vi "VI Tree.vi"   [LabVIEW 2018, in "Agilent PSG MXG Series.lvlib"]
doc: "This is the instrument driver for the Agilent PSG MXG Series. The VI Tree displays all the user-callable VIs of the instrument driver in an organized table."
uses:
  Agilent PSG MXG Series.lvlib
  Configure/Modulation/Configure Modulation (Amplitude).vi
  Configure/Modulation/Configure Modulation Waveform (Noise).vi
  Configure/Configure Sweep (List).vi
  Configure/Modulation/Configure Modulation Waveform Advanced (Swept-Sine).vi
  Action-Status/Load and Save Data (Generic Data).vi
  Action-Status/Query Waveform Completed (Dual ARB).vi
panel:
  # "(c) 2007-2016 National Instruments.  ALL RIGHTS RESERVED."
  # "SEE DIAGRAM\nFOR VI TREE."
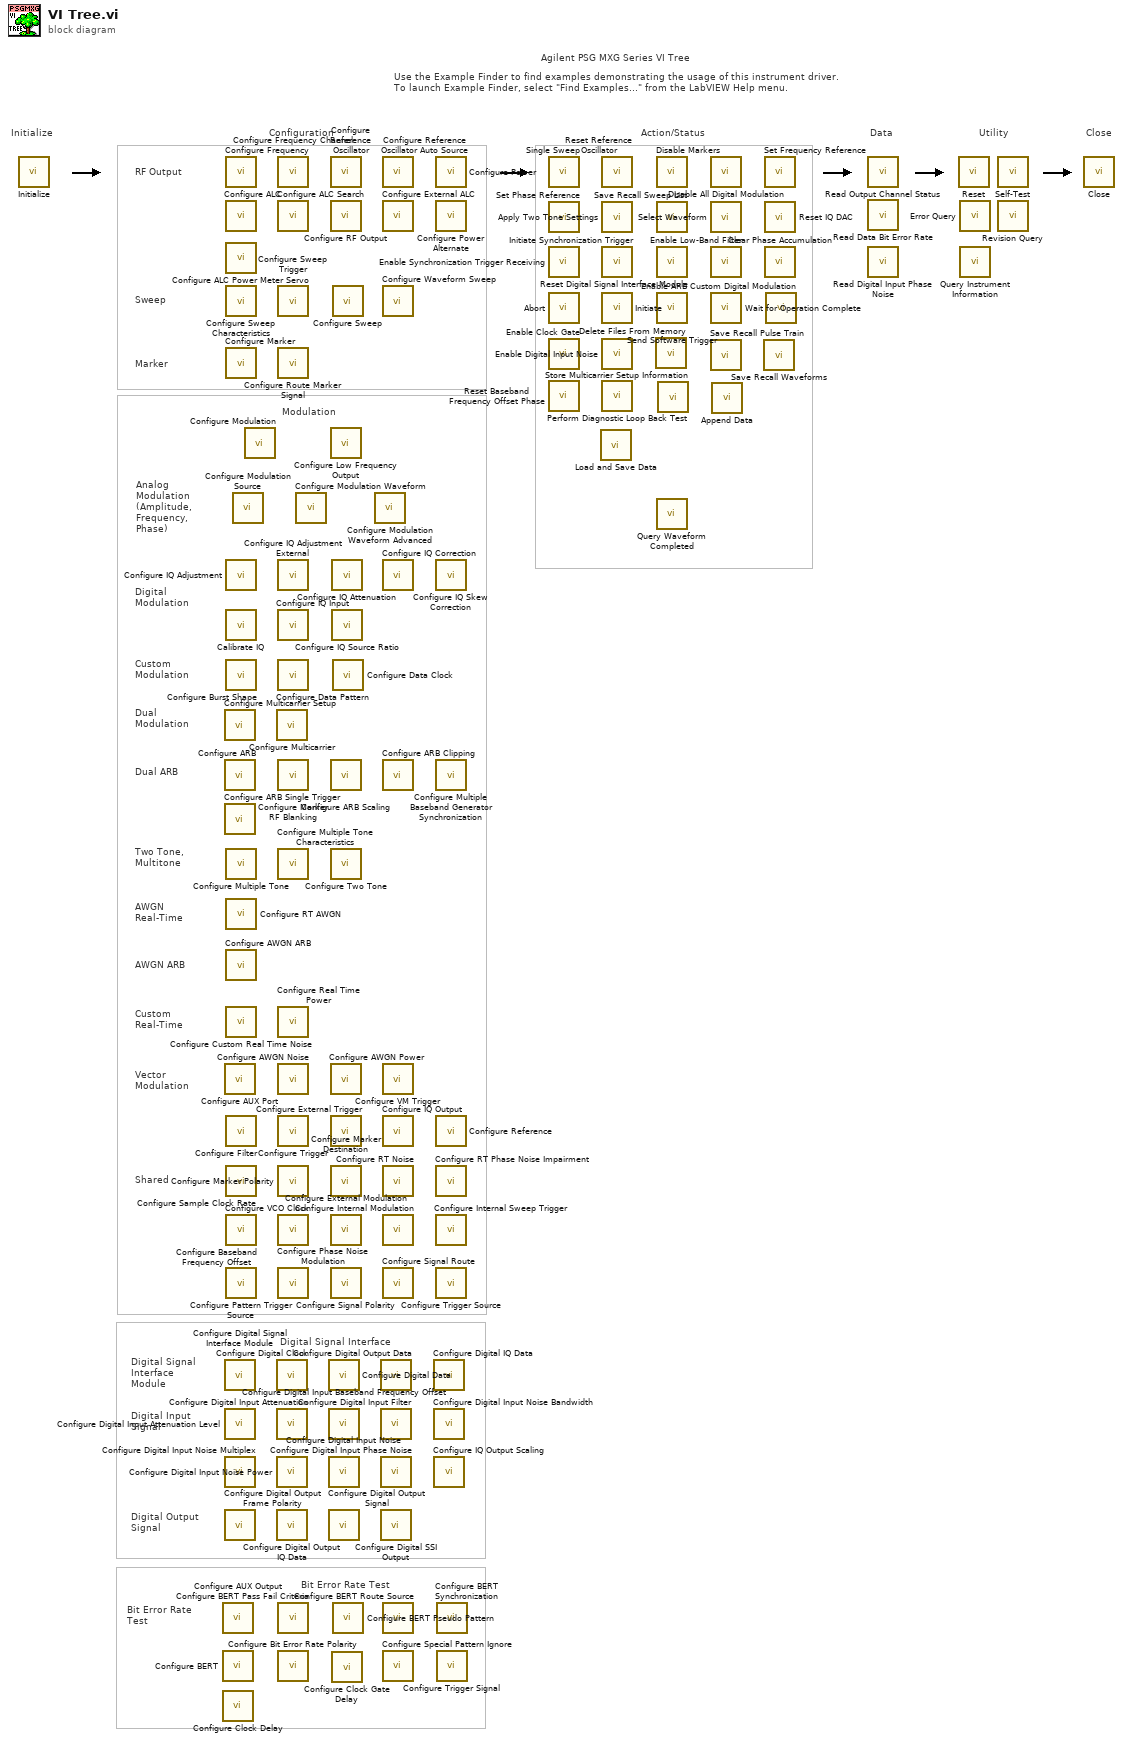
[diagram p0: block diagram]
diagram:
  # "Bit Error Rate Test"
  # "Bit Error Rate \nTest"
  # "Digital Output \nSignal"
  # "Digital Input \nSignal"
  # "Data"
  # "Vector\nModulation"
  # "Custom\nReal-Time"
  # "AWGN ARB"
  # "Digital Signal Interface"
  # "Marker"
  # "Digital Signal\nInterface\nModule"
  # "AWGN\nReal-Time"
  # "Shared"
  # "Two Tone,\nMultitone"
  # "Dual ARB"
  # "Dual\nModulation"
  # "Custom\nModulation"
  # "Digital\nModulation"
  # "Analog\nModulation\n(Amplitude,\nFrequency,\nPhase)"
  # "Sweep"
  # "RF Output"
  # "Modulation"
  # "Agilent PSG MXG Series VI Tree"
  # "Use the Example Finder to find examples demonstrating the usage of this instrument driver.\nTo launch Example Finder, select \"Find Examples...\" from the LabVIEW Help menu."
  # "Configuration"
  # "Utility"
  # "Action/Status"
  # "Close"
  # "Initialize"
  n1 = call "Initialize.vi"() -> ()  [unwired: 10 in, 2 out]
  n2 = call "Configure AUX Output.vi"() -> ()  [unwired: 10 in, 2 out]
  n3 = call "Configure BERT.vi"() -> ()  [unwired: 10 in, 2 out]
  n4 = call "Configure Clock Delay.vi"() -> ()  [unwired: 10 in, 2 out]
  n5 = call "Configure Multicarrier Setup.vi"() -> ()  [unwired: 14 in, 2 out]
  n6 = call "Configure ARB.vi"() -> ()  [unwired: 10 in, 2 out]
  n7 = call "Configure ARB Single Trigger.vi"() -> ()  [unwired: 10 in, 2 out]
  n8 = call "Configure AUX Port.vi"() -> ()  [unwired: 10 in, 2 out]
  n9 = call "Configure Digital Signal Interface Module.vi"() -> ()  [unwired: 10 in, 2 out]
  n10 = call "Configure Digital Input Attenuation Level.vi"() -> ()  [unwired: 10 in, 2 out]
  n11 = call "Configure Digital Input Noise Multiplex.vi"() -> ()  [unwired: 10 in, 2 out]
  n12 = call "Configure Digital Output Frame Polarity.vi"() -> ()  [unwired: 10 in, 2 out]
  n13 = call "Configure Frequency.vi"() -> ()  [unwired: 14 in, 2 out]
  n14 = call "Configure ALC.vi"() -> ()  [unwired: 14 in, 2 out]
  n15 = call "Configure ALC Power Meter Servo.vi"() -> ()  [unwired: 14 in, 2 out]
  n16 = call "Configure Sweep Characteristics.vi"() -> ()  [unwired: 14 in, 2 out]
  n17 = call "Configure Marker.vi"() -> ()  [unwired: 14 in, 2 out]
  n18 = call "Configure IQ Adjustment.vi"() -> ()  [unwired: 14 in, 2 out]
  n19 = call "Calibrate IQ.vi"() -> ()  [unwired: 10 in, 2 out]
  n20 = call "Configure Burst Shape.vi"() -> ()  [unwired: 14 in, 2 out]
  n21 = call "Configure Multiple Tone.vi"() -> ()  [unwired: 14 in, 2 out]
  n22 = call "Configure RT AWGN.vi"() -> ()  [unwired: 10 in, 2 out]
  n23 = call "Configure AWGN ARB.vi"() -> ()  [unwired: 10 in, 2 out]
  n24 = call "Configure Custom Real Time Noise.vi"() -> ()  [unwired: 10 in, 2 out]
  n25 = call "Configure Filter.vi"() -> ()  [unwired: 14 in, 2 out]
  n26 = call "Configure Sample Clock Rate.vi"() -> ()  [unwired: 10 in, 2 out]
  n27 = call "Configure Baseband Frequency Offset.vi"() -> ()  [unwired: 10 in, 2 out]
  n28 = call "Configure Pattern Trigger Source.vi"() -> ()  [unwired: 10 in, 2 out]
  n29 = call "Configure Modulation Source.vi"() -> ()  [unwired: 14 in, 2 out]
  n30 = call-poly "Configure Modulation.vi"() -> ()  [unwired: 14 in, 2 out]
  n31 = call "Configure Multicarrier.vi"() -> ()  [unwired: 10 in, 2 out]
  n32 = call "Configure Digital Clock.vi"() -> ()  [unwired: 14 in, 2 out]
  n33 = call "Configure Digital Input Attenuation.vi"() -> ()  [unwired: 10 in, 2 out]
  n34 = call "Configure Digital Input Noise Power.vi"() -> ()  [unwired: 10 in, 2 out]
  n35 = call "Configure Digital Output IQ Data.vi"() -> ()  [unwired: 10 in, 2 out]
  n36 = call "Configure Frequency Channel.vi"() -> ()  [unwired: 10 in, 2 out]
  n37 = call "Configure ALC Search.vi"() -> ()  [unwired: 14 in, 2 out]
  n38 = call "Configure Sweep Trigger.vi"() -> ()  [unwired: 14 in, 2 out]
  n39 = call "Configure Route Marker Signal.vi"() -> ()  [unwired: 10 in, 2 out]
  n40 = call "Configure IQ Adjustment External.vi"() -> ()  [unwired: 14 in, 2 out]
  n41 = call "Configure IQ Input.vi"() -> ()  [unwired: 10 in, 2 out]
  n42 = call "Configure Data Pattern.vi"() -> ()  [unwired: 10 in, 2 out]
  n43 = call "Configure Marker RF Blanking.vi"() -> ()  [unwired: 10 in, 2 out]
  n44 = call "Configure Multiple Tone Characteristics.vi"() -> ()  [unwired: 10 in, 2 out]
  n45 = call "Configure Real Time Power.vi"() -> ()  [unwired: 10 in, 2 out]
  n46 = call "Configure AWGN Noise.vi"() -> ()  [unwired: 14 in, 2 out]
  n47 = call "Configure Trigger.vi"() -> ()  [unwired: 14 in, 2 out]
  n48 = call "Configure Marker Polarity.vi"() -> ()  [unwired: 10 in, 2 out]
  n49 = call "Configure VCO Clock.vi"() -> ()  [unwired: 10 in, 2 out]
  n50 = call "Configure Phase Noise Modulation.vi"() -> ()  [unwired: 10 in, 2 out]
  n51 = call "Configure BERT Pass Fail Criteria.vi"() -> ()  [unwired: 10 in, 2 out]
  n52 = call "Configure Bit Error Rate Polarity.vi"() -> ()  [unwired: 10 in, 2 out]
  n53 = call-poly "Configure Modulation Waveform.vi"() -> ()  [unwired: 10 in, 2 out]
  n54 = call "Configure Digital Data.vi"() -> ()  [unwired: 14 in, 2 out]
  n55 = call "Configure Digital Input Baseband Frequency Offset.vi"() -> ()  [unwired: 10 in, 2 out]
  n56 = call "Configure Digital Input Noise.vi"() -> ()  [unwired: 10 in, 2 out]
  n57 = call "Configure Digital Output Signal.vi"() -> ()  [unwired: 10 in, 2 out]
  n58 = call "Configure Reference Oscillator.vi"() -> ()  [unwired: 10 in, 2 out]
  n59 = call "Configure RF Output.vi"() -> ()  [unwired: 10 in, 2 out]
  n60 = call "Configure Low Frequency Output.vi"() -> ()  [unwired: 14 in, 2 out]
  n61 = call "Configure ARB Scaling.vi"() -> ()  [unwired: 10 in, 2 out]
  n62 = call "Configure Two Tone.vi"() -> ()  [unwired: 10 in, 2 out]
  n63 = call "Configure AWGN Power.vi"() -> ()  [unwired: 10 in, 2 out]
  n64 = call "Configure External Trigger.vi"() -> ()  [unwired: 10 in, 2 out]
  n65 = call "Configure Marker Destination.vi"() -> ()  [unwired: 10 in, 2 out]
  n66 = call "Configure External Modulation.vi"() -> ()  [unwired: 10 in, 2 out]
  n67 = call "Configure Signal Polarity.vi"() -> ()  [unwired: 10 in, 2 out]
  n68 = call "Configure IQ Attenuation.vi"() -> ()  [unwired: 10 in, 2 out]
  n69 = call "Configure IQ Source Ratio.vi"() -> ()  [unwired: 10 in, 2 out]
  n70 = call "Configure Clock Gate Delay.vi"() -> ()  [unwired: 10 in, 2 out]
  n71 = call-poly "Configure Sweep.vi"() -> ()  [unwired: 14 in, 2 out]
  n72 = call "Configure Data Clock.vi"() -> ()  [unwired: 10 in, 2 out]
  n73 = call "Configure BERT Pseudo Pattern.vi"() -> ()  [unwired: 10 in, 2 out]
  n74 = call-poly "Configure Modulation Waveform Advanced.vi"() -> ()  [unwired: 14 in, 2 out]
  n75 = call "Configure Digital Output Data.vi"() -> ()  [unwired: 10 in, 2 out]
  n76 = call "Configure Digital Input Filter.vi"() -> ()  [unwired: 10 in, 2 out]
  n77 = call "Configure Digital Input Phase Noise.vi"() -> ()  [unwired: 10 in, 2 out]
  n78 = call "Configure Digital SSI Output.vi"() -> ()  [unwired: 10 in, 2 out]
  n79 = call "Configure Reference Oscillator Auto Source.vi"() -> ()  [unwired: 10 in, 2 out]
  n80 = call "Configure External ALC.vi"() -> ()  [unwired: 10 in, 2 out]
  n81 = call "Configure Waveform Sweep.vi"() -> ()  [unwired: 10 in, 2 out]
  n82 = call "Configure IQ Correction.vi"() -> ()  [unwired: 10 in, 2 out]
  n83 = call "Configure ARB Clipping.vi"() -> ()  [unwired: 10 in, 2 out]
  n84 = call "Configure VM Trigger.vi"() -> ()  [unwired: 10 in, 2 out]
  n85 = call "Configure IQ Output.vi"() -> ()  [unwired: 14 in, 2 out]
  n86 = call "Configure RT Noise.vi"() -> ()  [unwired: 14 in, 2 out]
  n87 = call "Configure Internal Modulation.vi"() -> ()  [unwired: 14 in, 2 out]
  n88 = call "Configure Signal Route.vi"() -> ()  [unwired: 10 in, 2 out]
  n89 = call "Configure BERT Route Source.vi"() -> ()  [unwired: 10 in, 2 out]
  n90 = call "Configure Special Pattern Ignore.vi"() -> ()  [unwired: 10 in, 2 out]
  n91 = call "Configure Digital IQ Data.vi"() -> ()  [unwired: 14 in, 2 out]
  n92 = call "Configure Digital Input Noise Bandwidth.vi"() -> ()  [unwired: 10 in, 2 out]
  n93 = call "Configure IQ Output Scaling.vi"() -> ()  [unwired: 10 in, 2 out]
  n94 = call "Configure Power.vi"() -> ()  [unwired: 14 in, 2 out]
  n95 = call "Configure Power Alternate.vi"() -> ()  [unwired: 10 in, 2 out]
  n96 = call "Configure IQ Skew Correction.vi"() -> ()  [unwired: 10 in, 2 out]
  n97 = call "Configure Multiple Baseband Generator Synchronization.vi"() -> ()  [unwired: 10 in, 2 out]
  n98 = call "Configure Reference.vi"() -> ()  [unwired: 10 in, 2 out]
  n99 = call "Configure RT Phase Noise Impairment.vi"() -> ()  [unwired: 10 in, 2 out]
  n100 = call "Configure Internal Sweep Trigger.vi"() -> ()  [unwired: 14 in, 2 out]
  n101 = call "Configure Trigger Source.vi"() -> ()  [unwired: 10 in, 2 out]
  n102 = call "Configure BERT Synchronization.vi"() -> ()  [unwired: 10 in, 2 out]
  n103 = call "Configure Trigger Signal.vi"() -> ()  [unwired: 14 in, 2 out]
  n104 = call "Single Sweep.vi"() -> ()  [unwired: 10 in, 2 out]
  n105 = call "Set Phase Reference.vi"() -> ()  [unwired: 10 in, 2 out]
  n106 = call "Enable Synchronization Trigger Receiving.vi"() -> ()  [unwired: 10 in, 2 out]
  n107 = call "Abort.vi"() -> ()  [unwired: 10 in, 2 out]
  n108 = call "Enable Clock Gate.vi"() -> ()  [unwired: 10 in, 2 out]
  n109 = call "Reset Baseband Frequency Offset Phase.vi"() -> ()  [unwired: 10 in, 2 out]
  n110 = call-poly "Load and Save Data.vi"() -> ()  [unwired: 14 in, 2 out]
  n111 = call "Reset Reference Oscillator.vi"() -> ()  [unwired: 10 in, 2 out]
  n112 = call "Apply Two Tone Settings.vi"() -> ()  [unwired: 10 in, 2 out]
  n113 = call "Initiate Synchronization Trigger.vi"() -> ()  [unwired: 10 in, 2 out]
  n114 = call "Initiate.vi"() -> ()  [unwired: 10 in, 2 out]
  n115 = call "Enable Digital Input Noise.vi"() -> ()  [unwired: 10 in, 2 out]
  n116 = call "Perform Diagnostic Loop Back Test.vi"() -> ()  [unwired: 9 in, 3 out]
  n117 = call "Delete Files From Memory.vi"() -> ()  [unwired: 10 in, 2 out]
  n118 = call "Disable Markers.vi"() -> ()  [unwired: 10 in, 2 out]
  n119 = call "Save Recall Sweep List.vi"() -> ()  [unwired: 10 in, 2 out]
  n120 = call "Reset Digital Signal Interface Module.vi"() -> ()  [unwired: 10 in, 2 out]
  n121 = call "Send Software Trigger.vi"() -> ()  [unwired: 10 in, 2 out]
  n122 = call-poly "Query Waveform Completed.vi"() -> ()  [unwired: 9 in, 3 out]
  n123 = call "Store Multicarrier Setup Information.vi"() -> ()  [unwired: 10 in, 2 out]
  n124 = call "Disable All Digital Modulation.vi"() -> ()  [unwired: 10 in, 2 out]
  n125 = call "Select Waveform.vi"() -> ()  [unwired: 10 in, 2 out]
  n126 = call "Enable Low-Band Filter.vi"() -> ()  [unwired: 10 in, 2 out]
  n127 = call "Wait for Operation Complete.vi"() -> ()  [unwired: 10 in, 2 out]
  n128 = call "Save Recall Pulse Train.vi"() -> ()  [unwired: 10 in, 2 out]
  n129 = call "Append Data.vi"() -> ()  [unwired: 10 in, 2 out]
  n130 = call "Save Recall Waveforms.vi"() -> ()  [unwired: 10 in, 2 out]
  n131 = call "Set Frequency Reference.vi"() -> ()  [unwired: 10 in, 2 out]
  n132 = call "Reset IQ DAC.vi"() -> ()  [unwired: 10 in, 2 out]
  n133 = call "Clear Phase Accumulation.vi"() -> ()  [unwired: 10 in, 2 out]
  n134 = call "Enable ARB Custom Digital Modulation.vi"() -> ()  [unwired: 10 in, 2 out]
  n135 = call "Read Output Channel Status.vi"() -> ()  [unwired: 9 in, 3 out]
  n136 = call "Read Data Bit Error Rate.vi"() -> ()  [unwired: 8 in, 4 out]
  n137 = call "Read Digital Input Phase Noise.vi"() -> ()  [unwired: 10 in, 6 out]
  n138 = call "Reset.vi"() -> ()  [unwired: 10 in, 2 out]
  n139 = call "Error Query.vi"() -> ()  [unwired: 8 in, 4 out]
  n140 = call "Query Instrument Information.vi"() -> ()  [unwired: 8 in, 8 out]
  n141 = call "Self-Test.vi"() -> ()  [unwired: 8 in, 4 out]
  n142 = call "Revision Query.vi"() -> ()  [unwired: 8 in, 4 out]
  n143 = call "Close.vi"() -> ()  [unwired: 11 in, 1 out]
